vi "EditorInterface.vi"() -> ()   [LabVIEW 2023]
uses:
  2025ReefBot/NewAuto/NewAutoStepTypedef.ctl
  2025ReefBot/NewAuto/NewAutoStepTypeEnum.ctl
  <vilib>/Rock Robotics/WPI/ThirdParty/JAS_Junk/TrajLib/Trajectory_Library.lvlib
panel:
  in  "write":bool
  in  "read":bool
  in  "Comment":string
  in  "Path":path
  in  "Array":T1[](array[typedef])
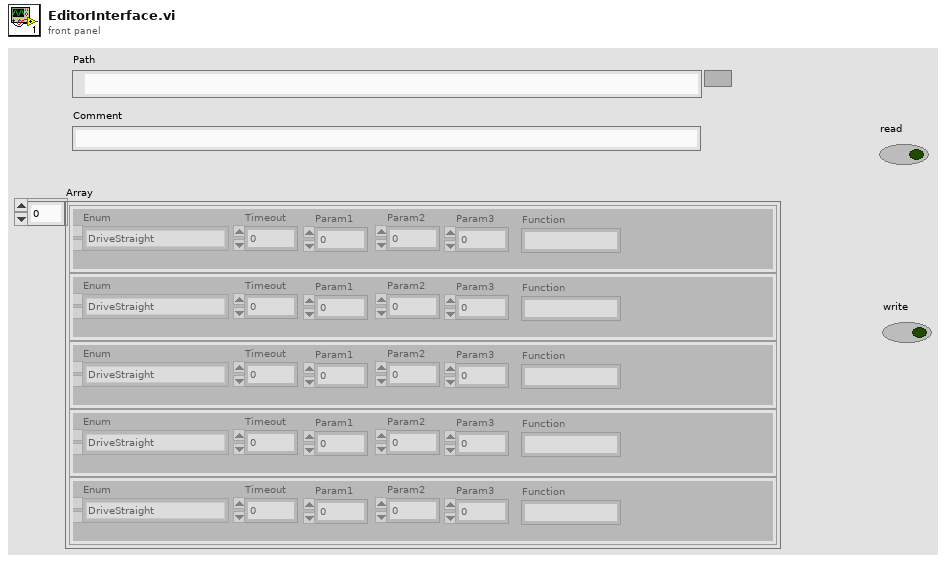
[diagram p1: front panel]
types:
  T1 = typedef "NewAutoStepTypedef.ctl" = cluster{"Enum":T2, "Timeout":dbl, "Param1":dbl, "Param2":dbl, "Param3":dbl, "Function":string}
  T2 = typedef "NewAutoStepTypeEnum.ctl" = enum16{"DriveStraight", "DriveTurn", "FollowAbsoluteTrajectory", "FollowRelativeTrajectory", "AutoWait", "ElevToRest", "ElevToFloor", "ElevToSource", "ElevToL1", "ElevToL2", "ElevToL3", "ElevToL4", "ElevToAlgae1", "ElevToAlgae2", "ElevToBarge", "ElevCancel", "IntakeCoral", "IntakeAlgae", "IntakeDepositCoral", "IntakeDepositAlgae", "IntakeCancel", "ElevRestWait", "ElevFloorWait", "ElevSourceWait", "ElevL1Wait", "ElevL2Wait", "ElevAlgae1Wait", "ElevL3Wait", "ElevAlgae2Wait", "ElevL4Wait", "ElevBargeWait"}
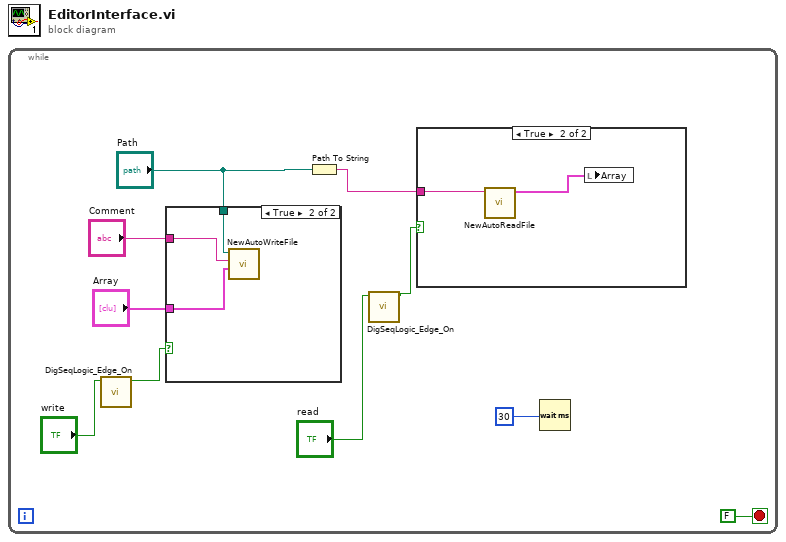
[diagram p0: block diagram]
diagram:
  n1 = while {
    stop <- FALSE stop-if-true
    n2 = call <vilib>:"DigSeqLogic_Edge_On.vi"("Input"="write") -> ("On Edge"=w4:bool)  [unwired: 10 in]
    n3 = case shown="True" w4 {
      tunnel: "Array" -> [_ w13]
      tunnel: "Comment" -> [_ w12]
      tunnel: "Path" -> [_ w11]
      frame False {
      }
      frame True {
        n4 = call "NewAutoWriteFile.vi"("Array"=w13, "Comment"=w12, "Trajectory File Name"=w11) -> ()  [unwired: 8 in, 1 out]
      }
    }
    n5 = Path To String(path="Path") -> (string=w10:string)
    n6 = call <vilib>:"DigSeqLogic_Edge_On.vi"("Input"="read") -> ("On Edge"=w5:bool)  [unwired: 10 in]
    n7 = case shown="True" w5 {
      tunnel: w10 -> [_ w15]
      frame False {
      }
      frame True {
        n8 = call "NewAutoReadFile.vi"("FileName"=w15) -> ("outTRAJECTORY"=w14:T1[])  [unwired: 8 in, 2 out]
        n9 = local write "Array"(w14) -> ()
      }
    }
    n10 = Wait (ms)(milliseconds to wait=u32 30 ("millisecond timer value")) -> ()  [unwired: 1 out]
  }
